vi "Get micronGrpc_MessageReply.vi"(8 "error in (no error)":errorcluster, 11 "gRPCid":T1) -> (0 "error out":errorcluster, 2 "package_templatemessage":T2, 3 "gRPCid out":T1)   [LabVIEW 2019, in "MicronGRPCGeneratedServer.lvlib"]
uses:
  MicronGRPCGeneratedServer.lvlib
  micronGrpc_MessageReply.ctl
  micronGrpc_MessageReply_Status.ctl
  <vilib>/gRPC/LabVIEW gRPC Library/Shared/grpcId.ctl
  micronGrpc_MessageReply_Flat.ctl
  micronGrpc_MessageReply_Status_Flat.ctl
  2ed25e12-861d-4677-8ead-ace2906b2041.vi
  <vilib>/gRPC/LabVIEW gRPC Library/Shared/TranslateGrpcError.vi
  FlatToRichmicronGrpc_MessageReply_Status.vi
  <vilib>/gRPC/LabVIEW gRPC Library/Server API/Server/Get Server DLL Path.vi
  <vilib>/Utility/error.llb/Error Cluster From Error Code.vi
  <vilib>/gRPC/LabVIEW gRPC Library/grpc-lvsupport-release.lvlib
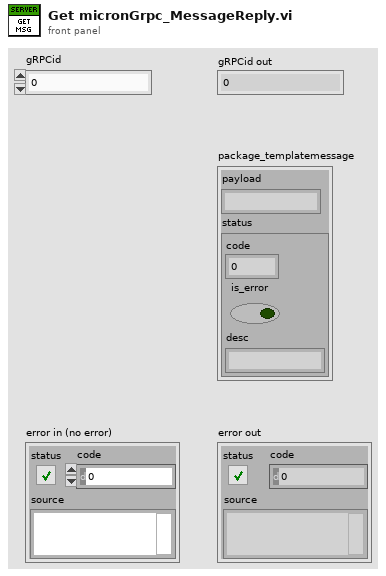
[diagram p1: front panel]
types:
  T1 = typedef "grpc-lvsupport-release.lvlib/grpcId.ctl" = u64
  T2 = typedef "MicronGRPCGeneratedServer.lvlib/micronGrpc_MessageReply.ctl" = cluster{"payload":string, "status":T3}
  T3 = typedef "MicronGRPCGeneratedServer.lvlib/micronGrpc_MessageReply_Status.ctl" = cluster{"code":i32, "is_error":bool, "desc":string}
  T4 = typedef "MicronGRPCGeneratedServer.lvlib/micronGrpc_MessageReply_Flat.ctl" = cluster{"payload":string, "status":T5}
  T5 = typedef "MicronGRPCGeneratedServer.lvlib/micronGrpc_MessageReply_Status_Flat.ctl" = cluster{"code":i32, "is_error":bool, "desc":string}
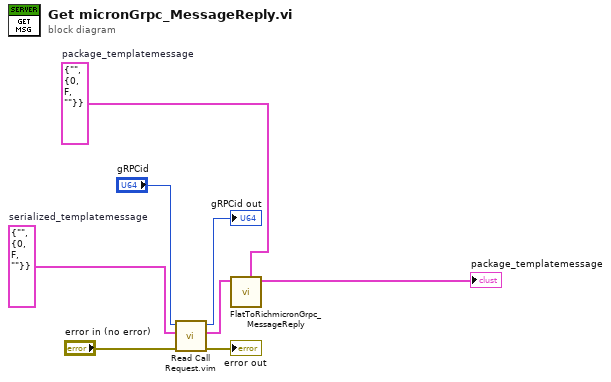
[diagram p0: block diagram]
diagram:
  w6 = T4 {"payload"="", "status"={"code"=0, "is_error"=FALSE, "desc"=""}}  # serialized_templatemessage
  w5 = T2 {"payload"="", "status"={"code"=0, "is_error"=FALSE, "desc"=""}}  # package_templatemessage
  n1 = call "Read Call Request.vim"("error in"="error in (no error)", "Request Type"=w6, "gRPCid in"="gRPCid") -> ("error out"=→"error out":errorcluster, "Request Data"=w4:T4, "gRPCid out"=→"gRPCid out":T1)  [unwired: 6 in]
  n2 = call "FlatToRichmicronGrpc_MessageReply.vi"("OutputClusterType"=w5, "InputCluster"=w4) -> ("OutputCluster"=→"package_templatemessage":T2)  [unwired: 9 in]
